vi "_Process Peaks.vi"(4 "X Step":dbl=1.0, 5 "Masses":dbl[](array[numeric]), 6 "Smoothed Data":dbl[](array[numeric]), 7 "Original Data":dbl[](array[numeric]), 8 "Peak List in":T1[](array[typedef])) -> (3 "Peak List out":T1[](array[typedef]))   [LabVIEW 2015]
uses:
  Type/_Peak Property.ctl
  <vilib>/Analysis/NI_AALBase.lvlib
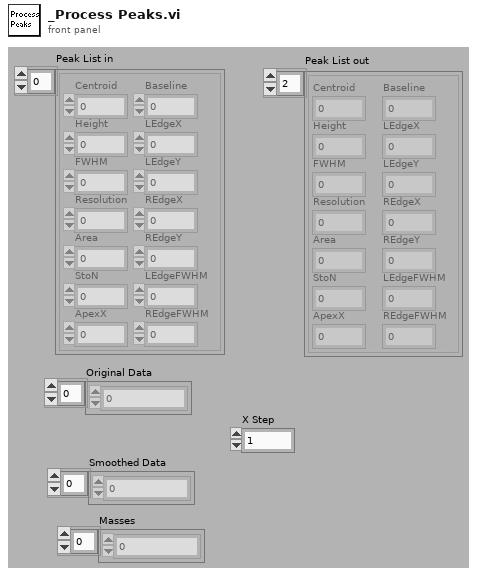
[diagram p1: front panel]
types:
  T1 = typedef "_Peak Property.ctl" = cluster{"Centroid":dbl, "Height":dbl, "FWHM":dbl, "Resolution":dbl, "Area":dbl, "StoN":dbl, "ApexX":dbl, "Baseline":dbl, "LEdgeX":dbl, "LEdgeY":dbl, "REdgeX":dbl, "REdgeY":dbl, "LEdgeFWHM":dbl, "REdgeFWHM":dbl}
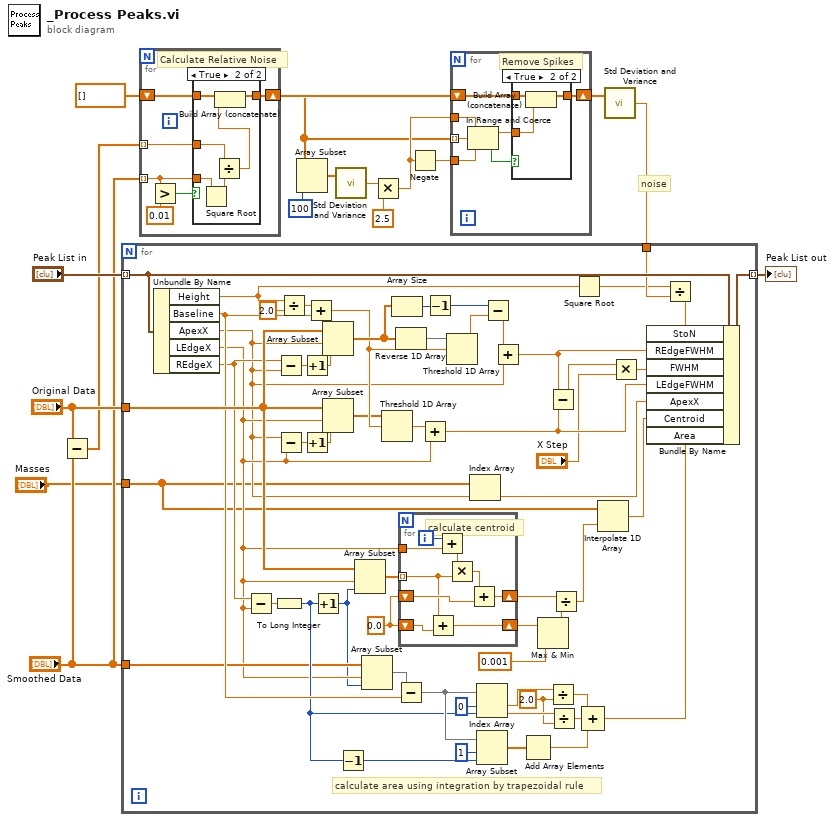
[diagram p0: block diagram]
diagram:
  w5 = dbl[] []
  # "noise"
  n1 = Subtract(x="Original Data", y="Smoothed Data") -> (x-y=w13:dbl[])
  n2 = for {
    tunnel: "Smoothed Data" -> [w19] mode=indexing
    tunnel: w13 -> [w22] mode=indexing
    shift-right: [w20] -> w4
    shift-left: w5 -> [w21]
    # "Calculate Relative Noise"
    n3 = Greater?(x=w19, y=0.01) -> (0:w17:bool)
    n4 = case shown="True" w17 {
      tunnel: w19 -> [_ w28]
      tunnel: w22 -> [_ w27]
      tunnel: w21 -> [w23 w26]
      tunnel: [w23 w24] -> w20
      frame False {
      }
      frame True {
        n5 = Square Root(x=w28) -> (sqrt(x)=w29:dbl)
        n6 = Divide(x=w27, y=w29) -> (x/y=w25:dbl)
        n7 = Build Array (concatenate)(w26, w25) -> (w24:dbl[])
      }
    }
  }
  n8 = Array Subset(array=w4, length=100) -> (w11:dbl[])  [unwired: 1 in]
  n9 = call <vilib>:"Std Deviation and Variance.vi"("X"=w11) -> ("standard deviation"=w8:dbl)  [unwired: 1 in, 2 out]
  n10 = Multiply(x=w8, y=2.5) -> (x*y=w6:dbl)
  n11 = Negate(x=w6) -> (-x=w7:dbl)
  n12 = for {
    tunnel: w4 -> [w34] mode=indexing
    shift-right: [w35] -> w3
    shift-left: w5 -> [w36]
    tunnel: w6 -> [w33]
    tunnel: w7 -> [w32]
    # "Remove Spikes"
    n13 = In Range and Coerce(upper limit=w33, x=w34, lower limit=w32) -> (coerced(x)=w30:dbl, In Range?=w31:bool)
    n14 = case shown="True" w31 {
      tunnel: w36 -> [w37 w40]
      tunnel: [w37 w39] -> w35
      tunnel: w30 -> [_ w38]
      frame False {
      }
      frame True {
        n15 = Build Array (concatenate)(w40, w38) -> (w39:dbl[])
      }
    }
  }
  n16 = call <vilib>:"Std Deviation and Variance.vi"("X"=w3) -> ("standard deviation"=w2:dbl)  [unwired: 1 in, 2 out]
  n17 = for {
    tunnel: "Peak List in" -> [w74] mode=indexing
    tunnel: [w72] -> w15 mode=indexing
    tunnel: "Original Data" -> [w73]
    tunnel: "Smoothed Data" -> [w56]
    tunnel: w2 -> [w47]
    tunnel: "Masses" -> [w42]
    w61 = 2.0 ("y")
    w95 = 0.0
    # "calculate area using integration by trapezoidal rule"
    n18 = Unbundle By Name(w74) -> ("Height"=w92:dbl, "Baseline"=w71:dbl, "ApexX"=w45:dbl, "LEdgeX"=w49:dbl, "REdgeX"=w57:dbl)
    n19 = Subtract(x=w57, y=w49) -> (x-y=w67:dbl)
    n20 = To Long Integer(number=w67) -> (32bit integer=w65:i32)
    n21 = Subtract(x=w57, y=w45) -> (x-y=w79:dbl)
    n22 = Subtract(x=w45, y=w49) -> (x-y=w78:dbl)
    n23 = Divide(x=w92, y=2.0) -> (x/y=w75:dbl)
    n24 = Increment(x=w79) -> (x+1=w80:dbl)
    n25 = Increment(x=w78) -> (x+1=w77:dbl)
    n26 = Add(x=w75, y=w71) -> (x+y=w82:dbl)
    n27 = Increment(x=w65) -> (x+1=w48:i32)
    n28 = Array Subset(array=w73, index=w45, length=w80) -> (w87:dbl[])
    n29 = Array Subset(array=w73, index=w49, length=w77) -> (w81:dbl[])
    n30 = Decrement(x=w65) -> (x-1=w66:i32)
    n31 = Array Subset(array=w73, index=w49, length=w48) -> (w50:dbl[])
    n32 = Array Subset(array=w56, index=w49, length=w48) -> (w55:dbl[])
    n33 = Threshold 1D Array(2:w82, 3:w81) -> (0:w83:dbl)  [unwired: 1 out]
    n34 = Array Size(array=w87) -> (size(s)=w88:i32)
    n35 = Reverse 1D Array(array=w87) -> (reversed array=w86:dbl[])
    n36 = Subtract(x=w55, y=w71) -> (x-y=w69:dbl[])
    n37 = for {
      tunnel: w50 -> [w101] mode=indexing
      shift-right: [w105] -> w94
      shift-left: w95 -> [w107]
      tunnel: w49 -> [w103]
      shift-right: [w99] -> w96
      shift-left: w95 -> [w100]
      i -> [w104]
      # "calculate centroid"
      n38 = Add(x=w101, y=w100) -> (x+y=w99:dbl)
      n39 = Add(x=w104, y=w103) -> (x+y=w102:dbl)
      n40 = Multiply(x=w102, y=w101) -> (x*y=w106:dbl)
      n41 = Add(x=w106, y=w107) -> (x+y=w105:dbl)
    }
    n42 = Add(x=w83, y=w49) -> (x+y=w85:dbl)
    n43 = Decrement(x=w88) -> (x-1=w91:i32)
    n44 = Threshold 1D Array(2:w82, 3:w86) -> (0:w89:dbl)  [unwired: 1 out]
    n45 = Index Array(array=w42, index=w45) -> (element=w44:dbl)
    n46 = Index Array(array=w69, index #1=0 ("index"), index #2=w65) -> (element #1=w63:dbl, element #2=w62:dbl)
    n47 = Array Subset(array=w69, index=1, length=w66) -> (w64:dbl[])
    n48 = Subtract(x=w91, y=w89) -> (x-y=w90:dbl)
    n49 = Add(x=w90, y=w45) -> (x+y=w84:dbl)
    n50 = Add Array Elements(numeric array=w64) -> (sum=w58:dbl)
    n51 = Max & Min(x=w96, y=0.001) -> (max(x,y)=w97:dbl)  [unwired: 1 out]
    n52 = Subtract(x=w84, y=w85) -> (x-y=w53:dbl)
    n53 = Divide(x=w63, y=w61) -> (x/y=w60:dbl)
    n54 = Divide(x=w62, y=w61) -> (x/y=w59:dbl)
    n55 = Divide(x=w94, y=w97) -> (x/y=w43:dbl)
    n56 = Square Root(x=w92) -> (sqrt(x)=w46:dbl)
    n57 = Compound Arithmetic op=ADD(w60, w59, w58) -> (w54:dbl)
    n58 = Interpolate 1D Array(1:w43, 2:w42) -> (0:w41:dbl)
    n59 = Multiply(x=w53, y="X Step") -> (x*y=w52:dbl)
    n60 = Divide(x=w46, y=w47) -> (x/y=w93:dbl)
    n61 = Bundle By Name(cluster=w74, "StoN"=w93, "REdgeFWHM"=w84, "FWHM"=w52, "LEdgeFWHM"=w85, "ApexX"=w44, "Centroid"=w41, "Area"=w54) -> (w72:T1)
  }
  "Peak List out" <- w15
